vi "Histogram Main.vi"() -> ()   [LabVIEW 2015]
uses:
  Consumer Message.ctl
  <vilib>/ErrorRing/Error Ring.xnode
panel:
  in  "signal":u16(ring) items=["uniform white", "uniform+uniform", "Gaussian white", "sine", "square"]
  out "Consumer Shutdown?":bool
  out "State to Execute":string
  out "High Priority?":bool
  out "Backlog":u8(slide) scale=0.0..100.0
  out "Processed Value":i32
  in  "High Priority Message":bool
  in  "Normal Priority Message":bool
  in  "Stop":bool
  # "Number of enqueued messages waiting to be processed"
  # "Current data being processed in consumer loop"
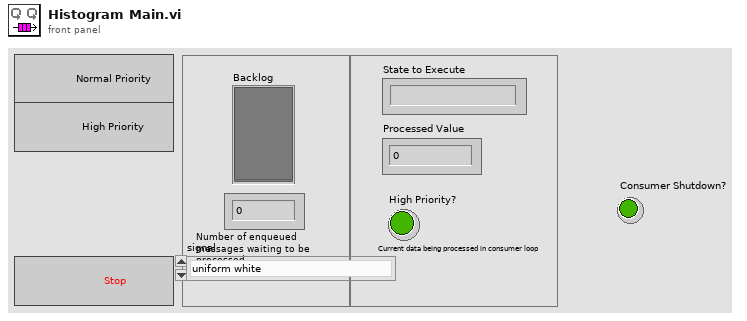
[diagram p1: front panel]
types:
  T1 = typedef "Consumer Message.ctl" = cluster{"Consumer State":string, "Boolean Data":bool, "Numeric Data":i32, "signal":dbl[], "Numeric":dbl, "Error":errorcluster}
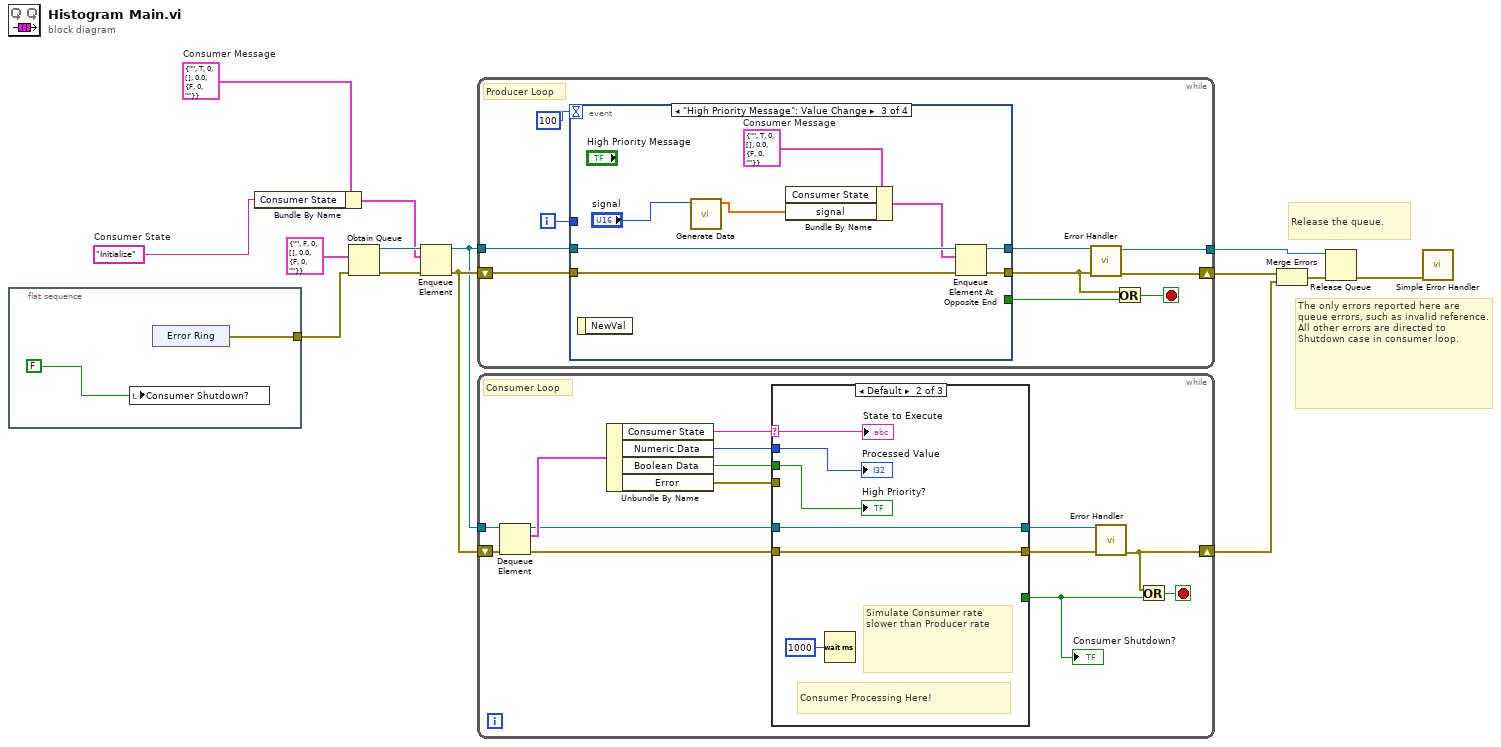
[diagram p0: block diagram]
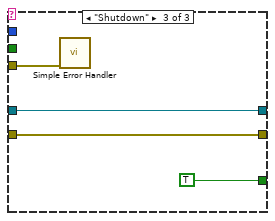
[diagram p3: hidden frame]
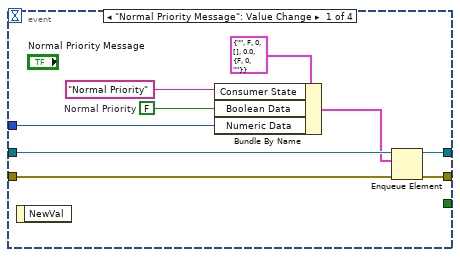
[diagram p4: hidden frame]
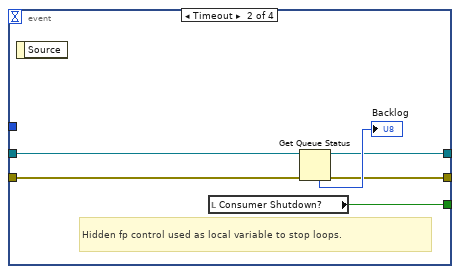
[diagram p5: hidden frame]
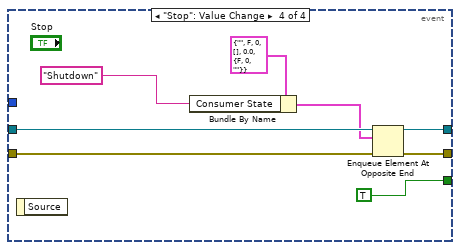
[diagram p6: hidden frame]
diagram:
  w6 = "Initialize"  # Consumer State
  w8 = T1 {"Consumer State"="", "Boolean Data"=TRUE, "Numeric Data"=0, "signal"=[], "Numeric"=0.0, "Error"={"status"=FALSE, "code"=0, "source"=""}}  # Consumer Message
  # "Release the queue."
  # "The only errors reported here are queue errors, such as invalid reference.  All other errors are directed to Shutdown case in consumer loop."
  n1 = flat-sequence {
    tunnel: [w15] -> w9
    frame #0 {
      n2 = local write "Consumer Shutdown?"(FALSE ("Stop Loops (local)")) -> ()
      n3 = xnode "Error Ring"() -> ("error out"=w15:errorcluster)
    }
  }
  n4 = Bundle By Name(cluster=w8, "Consumer State"=w6) -> (w7:T1)
  n5 = Obtain Queue(element data type=T1 {"Consumer State"="", "Boolean Data"=FALSE, "Numeric Data"=0, "signal"=[], "Numeric"=0.0, "Error"={"status"=FALSE, "code"=0, "source"=""}}, error in (no error)=w9) -> (queue out=w11:refnum<queue>, error out=w14:errorcluster)  [unwired: 3 in, 1 out]
  n6 = Enqueue Element(queue=w11, element=w7, error in (no error)=w14) -> (queue out=w10:refnum<queue>, error out=w12:errorcluster)  [unwired: 1 in, 1 out]
  n7 = while {
    tunnel: w10 -> [w27]
    shift-right: [w19] -> w5
    shift-left: w12 -> [w26]
    tunnel: [w18] -> w1
    i -> [w25]
    stop <- w21 stop-if-true
    # "Producer Loop"
    n8 = event shown="[2] \"High Priority Message\": Value Change" {
      selector: _ -> [_ _ _ _]
      dyn-events: _ -> [_ _ _ _]
      timeout: 100 -> [_ _ _ _]
      tunnel: w27 -> [w36 w40 w49 w58]
      tunnel: w26 -> [w34 w39 w48 w56]
      tunnel: [w35 w38 w50 w55] -> w20
      tunnel: [_ w42 _ TRUE] -> w22
      tunnel: w25 -> [w33 _ _ _]
      tunnel: [w29 w37 w46 w54] -> w24
      event "Normal Priority Message": Value Change {
        w30 = FALSE  # Normal Priority
        n9 = event-data() -> ()  [unwired: 1 in, 1 out]
        n10 = Bundle By Name(cluster=T1 {"Consumer State"="", "Boolean Data"=FALSE, "Numeric Data"=0, "signal"=[], "Numeric"=0.0, "Error"={"status"=FALSE, "code"=0, "source"=""}}, "Consumer State"="Normal Priority" ("String Data"), "Boolean Data"=w30, "Numeric Data"=w33) -> (w32:T1)
        n11 = Enqueue Element(queue=w36, element=w32, error in (no error)=w34) -> (queue out=w29:refnum<queue>, error out=w35:errorcluster)  [unwired: 1 in, 1 out]
      }
      event Timeout {
        # "Hidden fp control used as local variable to stop loops."
        n12 = event-data() -> ()  [unwired: 1 in, 1 out]
        n13 = local read "Consumer Shutdown?"() -> (w42:bool)
        n14 = Get Queue Status(queue=w40, error in (no error)=w39) -> (queue out=w37:refnum<queue>, error out=w38:errorcluster, # elements in queue=→"Backlog":i32)  [unwired: 1 in, 5 out]
      }
      event "High Priority Message": Value Change {
        w45 = T1 {"Consumer State"="", "Boolean Data"=TRUE, "Numeric Data"=0, "signal"=[], "Numeric"=0.0, "Error"={"status"=FALSE, "code"=0, "source"=""}}  # Consumer Message
        n15 = event-data() -> ()  [unwired: 1 in, 1 out]
        n16 = call "Generate Data.vi"("signal"="signal") -> ("Y"=w44:dbl[])  [unwired: 9 in, 1 out]
        n17 = Bundle By Name(cluster=w45, "signal"=w44) -> (w47:T1)  [unwired: 1 in]
        n18 = Enqueue Element At Opposite End(queue=w49, element=w47, error in (no error)=w48) -> (queue out=w46:refnum<queue>, error out=w50:errorcluster)  [unwired: 1 in, 1 out]
      }
      event "Stop": Value Change {
        n19 = event-data() -> ()  [unwired: 1 in, 1 out]
        n20 = Bundle By Name(cluster=T1 {"Consumer State"="", "Boolean Data"=FALSE, "Numeric Data"=0, "signal"=[], "Numeric"=0.0, "Error"={"status"=FALSE, "code"=0, "source"=""}}, "Consumer State"="Shutdown") -> (w51:T1)
        n21 = Enqueue Element At Opposite End(queue=w58, element=w51, error in (no error)=w56) -> (queue out=w54:refnum<queue>, error out=w55:errorcluster)  [unwired: 1 in, 1 out]
      }
    }
    n22 = call "Error Handler.vi"("error in"=w20, "queue in"=w24) -> ("error out"=w19:errorcluster, "queue out"=w18:refnum<queue>)  [unwired: 8 in]
    n23 = Or(x=w20, y=w22) -> (x .or. y?=w21:bool)
  }
  n24 = while {
    tunnel: w10 -> [w72]
    shift-right: [w61] -> w4
    shift-left: w12 -> [w71]
    stop <- w62 stop-if-true
    # "Consumer Loop"
    n25 = Dequeue Element(queue=w72, error in (no error)=w71) -> (queue out=w60:refnum<queue>, element=w70:T1, error out=w59:errorcluster)  [unwired: 1 in, 1 out]
    n26 = Unbundle By Name(w70) -> ("Consumer State"=w69:string, "Numeric Data"=w68:i32, "Boolean Data"=w67:bool, "Error"=w64:errorcluster)
    n27 = case shown="Default" w69 {
      selector: w69 -> [_ w77 _]
      tunnel: [_ _ TRUE] -> w63
      tunnel: w59 -> [w73 w75 w81]
      tunnel: [w73 w75 w81] -> w66
      tunnel: w68 -> [_ w80 _]
      tunnel: w67 -> [_ w79 _]
      tunnel: w60 -> [w74 w78 w82]
      tunnel: [w74 w78 w82] -> w65
      tunnel: w64 -> [_ _ w83]
      frame "Initialize" {
      }
      frame Default {
        # "Simulate Consumer rate slower than Producer rate"
        # "Consumer Processing Here!"
        n28 = Wait (ms)(milliseconds to wait=u32 1000) -> ()  [unwired: 1 out]
        "Processed Value" <- w80
        "High Priority?" <- w79
        "State to Execute" <- w77
      }
      frame "Shutdown" {
        n29 = call <vilib>:"Simple Error Handler.vi"("error in (no error)"=w83) -> ()  [unwired: 4 in, 5 out]
      }
    }
    "Consumer Shutdown?" <- w63
    n30 = call "Error Handler.vi"("error in"=w66, "queue in"=w65) -> ("error out"=w61:errorcluster)  [unwired: 8 in, 1 out]
    n31 = Or(x=w61, y=w63) -> (x .or. y?=w62:bool)
  }
  n32 = Merge Errors(w5, w4) -> (w3:errorcluster)
  n33 = Release Queue(queue=w1, error in (no error)=w3) -> (error out=w2:errorcluster)  [unwired: 1 in, 2 out]
  n34 = call <vilib>:"Simple Error Handler.vi"("error in (no error)"=w2) -> ()  [unwired: 4 in, 5 out]
